vi "AlliGator FLI Dataset Loading Core.vi"(4 "Data Description":string, 5 "Control References":T4, 6 "Metadata":string, 7 "Image Type":string, 8 "error in (no error)":errorcluster, 9 "FLI Data File Information":T1, 10 "selected path":path, 11 "Data Value Reference in":refnum<data-value>) -> (0 "error out":errorcluster, 2 "Message":string, 3 "Data Value Reference out":refnum<data-value>)   [LabVIEW 2021, in "AlliGator Files.lvlib"]
doc: "Core VI handling loading the multiple gate images of a dataset as well as associated information and metadata. It dynamically calls a dataset-specific set of VIs to perform the actual loading."
uses:
  AlliGator Files.lvlib
  AlliGator Dataset Ctrl Refnums.ctl
  AlliGator Displayed Image.ctl
  AlliGator FLI Data File Information.ctl
  Phasor/Phasor Fluorescence Lifetime Parameters v3.ctl
  AlliGator FLI Dataset Type.ctl
  AlliGator Internal Variables v2.ctl
  <vilib>/vision/Image Controls.llb/IMAQ Image.ctl
  AlliGator Gate Image Set.ctl
  AlliGator Data Series Type.ctl
  AlliGator Dataset Channel.ctl
  AlliGator Gate Arithmetic.ctl
  Image/Named ROI Description.ctl
  AlliGator Decay Metadata v3.ctl
  AlliGator Decay Background Subtraction Info.ctl
  AlliGator Baseline Subtraction Method.ctl
  Graphs/XY Graph/XY Graph Plot Shift Parameters.ctl
  Graphs/XY Graph/XY Graph Plot Shift Method.ctl
  AlliGator Decay Extrapolation Parameters.ctl
  Phasor/Calibration Phasor (m, phi).ctl
  Phasor/Phasor Reference Series.ctl
  Phasor/Phasor Calibration Map v2.ctl
  Phasor/Phasor (g, s).ctl
  AlliGator Raw Phasor Plot Data v4.ctl
  Phasor/Phasor Standard Deviation Options.ctl
  AlliGator Phasor Multi-Harmonic Data.ctl
  Phasor/Phasor Harmonic Data.ctl
  AlliGator Decay Fit Options & Parameters v2.ctl
  Fits/IRF(X)PSED/Decay Fit Options v2.ctl
  Fits/Decay Convolution/Decay Model.ctl
  Fits/Residual Type.ctl
  Fits/IRF(X)PSED/Fit Weights Type.ctl
  Fits/Non-linear Fitting Method v2.ctl
  Fits/Fit Calculation Method.ctl
  Fits/Non-linear Fitting Algorithm.ctl
  AlliGator Decay Fit Parameter Constraints 2.ctl
  Fits/IRF(X)PSED/Decay Fit Parameters In List.ctl
  Fits/IRF(X)PSED/MLE Baseline Offset Type.ctl
  AlliGator Decay Preprocessing Parameters.ctl
  Fits/IRF(X)PSED/Decay Fit Parameters & Derived Quantities List.ctl
  AlliGator Parameter Maps Data.ctl
  AlliGator Image Pre-processing Parameters.ctl
  Arrays/Kernel Type.ctl
  Arrays/Smoothing Algorithm.ctl
  SwissSPAD/SwissSPAD Live_Image Display Options.ctl
  AlliGator Image Pre-processing Step.ctl
  AlliGator FLI Image Stack Action.ctl
  AlliGator Variables List.ctl
  AlliGator After Loading Dataset Information.ctl
  AlliGator ICCD-specific Information.ctl
  AlliGator Source Image.lvlib
  AlliGator HDF5.lvlib
  Time/Time.lvlib
  Arrays/Arrays.lvlib
  Strings/Strings.lvlib
  AlliGator GUI.lvlib
  GUI/GUI.lvlib
  Error/Error.lvlib
  AlliGator Dual-Channel Datasets.lvlib
  Image/Image.lvlib
  SwissSPAD/SwissSPAD Live.lvlib
  AlliGator Globals, Variables & Constants.lvlib
  Files/Files.lvlib
  Phasor/Phasor.lvlib
  AlliGator Decay Preprocessing.lvlib
  Graphs/XY Graph/XY Graph Add-Ons.lvlib
  AlliGator Phasor Graph.lvlib
  AlliGator Phasor Plot.lvlib
  Fits/Fits.lvlib
  AlliGator Decay Fit.lvlib
  AlliGator Decay Fit Parameter Map.lvlib
  AlliGator Internal Variables.lvlib
  AlliGator Settings.lvlib
panel:
  out "Dual-Channel Dataset":bool
  out "# created images":i32
  out "# Disposed Images":i32
  # "see the AlliGator License on the block diagram (Ctrl+E or Window:Show Block Diagram)"
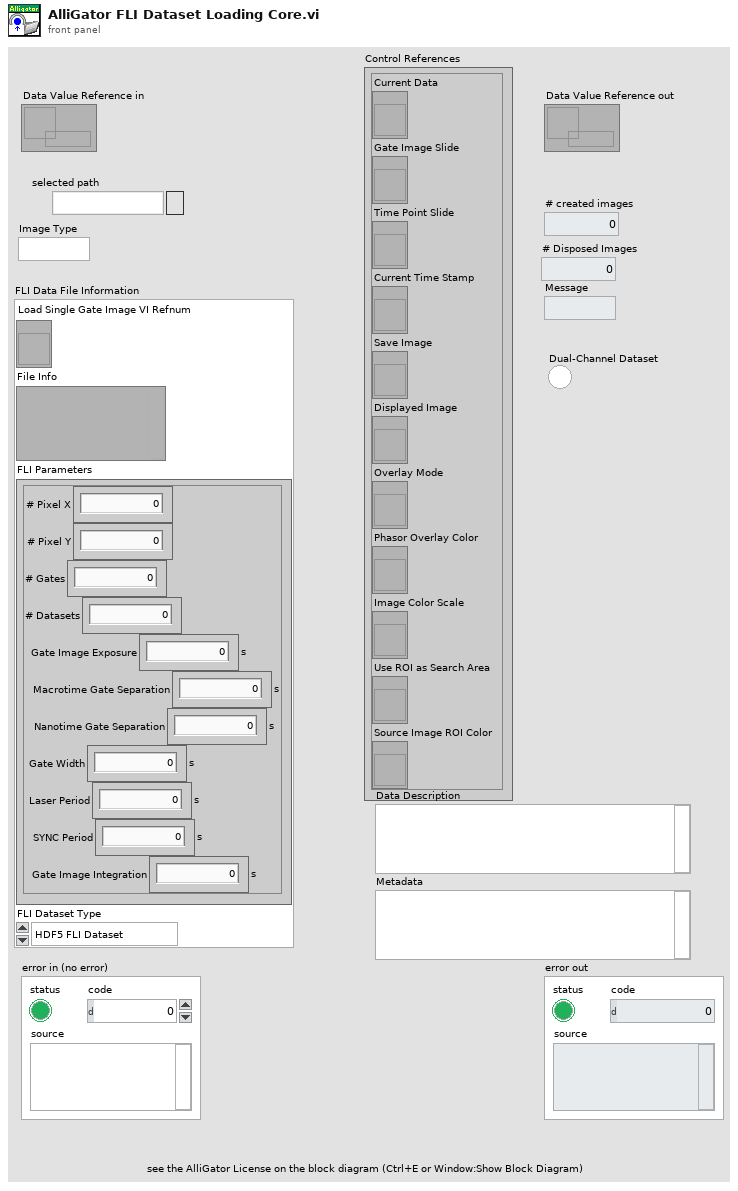
[diagram p1: front panel]
types:
  T1 = typedef "AlliGator HDF5.lvlib/AlliGator FLI Data File Information.ctl" = cluster{"Load Single Gate Image VI Refnum":refnum<vi>, "File Info":variant, "FLI Parameters":T2, "FLI Dataset Type":T3}
  T2 = typedef "Phasor.lvlib/Phasor Fluorescence Lifetime Parameters v3.ctl" = cluster{"# Pixel X":i32, "# Pixel Y":i32, "# Gates":i32, "# Datasets":i32, "Gate Image Exposure":dbl[unit], "Macrotime Gate Separation":dbl[unit], "Nanotime Gate Separation":dbl[unit], "Gate Width":dbl[unit], "Laser Period":dbl[unit], "SYNC Period":dbl[unit], "Gate Image Integration":dbl[unit]}
  T3 = typedef "AlliGator Files.lvlib/AlliGator FLI Dataset Type.ctl" = enum16{"HDF5 FLI Dataset", "Gate Image Folder", ".sdt FLI Dataset (Becker & Hickl)", ".ptu FLI Dataset (PicoQuant)", "SS1 FLI Dataset", "SS2 FLI Dataset", "I/m/phi Dataset", ".bin FLI Dataset (PicoQuant Binned)", ".bin FLI Dataset (Piccolo Binned)"}
  T4 = typedef "AlliGator GUI.lvlib/AlliGator Dataset Ctrl Refnums.ctl" = cluster{"Current Data":refnum<vi>, "Gate Image Slide":refnum<vi>, "Time Point Slide":refnum<vi>, "Current Time Stamp":refnum<vi>, "Save Image":refnum<vi>, "Displayed Image":refnum<vi>, "Overlay Mode":refnum<vi>, "Phasor Overlay Color":refnum<vi>, "Image Color Scale":refnum<vi>, "Use ROI as Search Area":refnum<vi>, "Source Image ROI Color":refnum<vi>}
  T5 = typedef "AlliGator Files.lvlib/AlliGator Image Pre-processing Parameters.ctl" = cluster{"Pile-up Correction":bool, "Pixel Well Capacity":u32, "Use Image Binning":bool, "X Bin":i32, "Y Bin":i32, "Use Image Smoothing":bool, "Kernel Type":T6, "Bin":i32, "Algorithm":T7, "Hot Pixel Removal":T8, "Dataset Scaling Factor":dbl, "Image Pre-processing Steps":T9[]}
  T6 = typedef "Arrays.lvlib/Kernel Type.ctl" = enum16{"Uniform", "Bilinear", "Gaussian"}
  T7 = typedef "Arrays.lvlib/Smoothing Algorithm.ctl" = enum16{"Rapid", "Thorough"}
  T8 = typedef "SwissSPAD Live.lvlib/SwissSPAD Live_Image Display Options.ctl" = cluster{"Remove Screamers":bool, "Delta":sgl, "Equalize Histogram":bool, "Percentile":sgl, "Hot Pixel Mask Image":path, "Use Hot Pixel Mask":bool}
  T9 = typedef "AlliGator Files.lvlib/AlliGator Image Pre-processing Step.ctl" = enum16{"Remove Screamers", "Pile-up Correction", "Binning", "Smoothing", "Rescaling", "Dead Left Column Correction"}
  T10 = typedef "AlliGator Source Image.lvlib/AlliGator Image Loading Options.ctl" = cluster{"Pixel Well Capacity":u32, "Pile-up Correction":bool, "Gate Step":i32, "Image Smoothing Options":T11, "Gates to Skip":T12, "File Background Subtraction":bool, "Background File Path":path, "Image Binning Options":T13, "# Gates":u32, "Gates to Keep":T14, "Define Gates to":bool, "Hot Pixel Removal":T8, "Dataset Scaling Factor":dbl, "Image Pre-processing Steps":T9[]}
  T11 = typedef "AlliGator Settings.lvlib/AlliGator Image Smoothing Options.ctl" = cluster{"Use Image Smoothing":bool, "Kernel Type":T6, "Bin":i32, "Algorithm":T7}
  T12 = typedef "AlliGator Decay Analysis.lvlib/AlliGator Gates to Skip.ctl" = cluster{"Start":u32, "End":u32}
  T13 = typedef "AlliGator Source Image.lvlib/AlliGator Image Binning Options.ctl" = cluster{"Use Image Binning":bool, "X Bin":i32, "Y Bin":i32}
  T14 = typedef "AlliGator Settings.lvlib/AlliGator Gates to Keep.ctl" = cluster{"First":u32, "Last":u32}
  T15 = typedef "AlliGator Settings.lvlib/AlliGator Gate Arithmetic.ctl" = enum16{"None", "INT-G2", "G2/INT*<INT>", "(1 - G2/INT)*<INT>"}
  T16 = typedef "AlliGator Dual-Channel Datasets.lvlib/AlliGator Dataset Channel.ctl" = enum16{"G2", "INT"}
  T17 = typedef "Image.lvlib/Image Characteristics.ctl" = cluster{"Calibration":T18, "File Type":string, "X Resolution":i32, "Y Resolution":i32, "File Data Type":i32, "Image Type":T20}
  T18 = typedef "Simple Grid Descriptor" = cluster{"X Step":sgl, "Y Step":sgl, "Unit":T19}
  T19 = typedef "Image Unit" = enum32{"Undefined", "Angström", "Micrometer", "Millimeter", "Centimeter", "Meter", "Kilometer", "Microinch", "Inch", "Feet", "Nautical miles", "Standard miles", "Steps"}
  T20 = typedef "Image Type" = u32
  T21 = typedef "AlliGator HDF5.lvlib/AlliGator FLI Image Stack Action.ctl" = enum16{"Init", "Get Image", "Close"}
  T22 = typedef "AlliGator Globals, Variables & Constants.lvlib/AlliGator Variables List.ctl" = enum16{"---- GUI ----", "GUI:Initialization Status", "GUI:State Indicators Refnum", "GUI:Original AlliGator Menu Items", "GUI:Current Action Loop State", "GUI:Script in progress", "GUI:Playback", "GUI:Loop Playback", "GUI:Search ROI Used", "GUI:Search ROI", "Decay Graph Max Legend Size", "Intensity Graph Max Legend Size", "Decay Statistics Graph Max Legend Size", "Phasor Graph Max Legend Size", "Phasor Ratio Graph Max Legend Size", "Lifetime Graph Max Legend Size", "---- Files ----", "Files:Export Dataset Frames as Individual Files", "Files:Show Batch Export Help Balloons", "Files:Frames in Dataset", "Files:ptu File Frame Start Indices", "Files:Current Frame in Dataset", "Files:Current Frame Timestamp", "Files:Dataset Loaded", "Files:Dataset Metadata", "Files:Dataset Channel", "Files:Dataset Data Description", "Files:Background Dataset Metadata", "Files:Background Dataset Channel", "Files:Background Dataset Data Description", "Files:Background File Subtraction", "Files:Background File Path", "Files:Background File Pile-up Correction", "Files:Background File Pixel Well Capacity", "Files:Background File Scaling Factor", "Files:Current Dataset Load Settings", "Files:Dataset Path", "Files:ICCD-specific Information", "Files:Macrotime Gate Separation", "------ Python Plugins ------", "Python Plugins:Information", "Python Plugins:Python Session", "Python Plugins:Valid Python Session?", "---- Source Image ----", "Source Image:ROIs", "Source Image:Current ROI", "Source Image:ROI Event Refnum", "X_Source Image Display Range", "X_Source Image Palette Information", "X_Type of Displayed Image", "X_Time Gate Slider", "Source Image:Palette List", "Source Image:Scale", "Source Image:ROI Overlay Color", "Source Image:Overlay to Erase", "Source Image:Is Displayed Image Accumulated", "Source Image:White Light Image Modified", "Source Image:Mask Image Modified", "---- Image Profile Window ----", "Image Profile:Window Event Refnum", "Image Profile:IntensityType", "Image Profile:Intensity Average Type", "Image Profile:Intensity-weighted SDV", "Image Profile:Box Profile Type", "Image Profile:Window Open", "Image Profile:Plotted Fit Parameter", "------ Phasor Graph -------", "Phasor Graph:Show Line", "---- Phasor Plot ---", "Phasor Plot:Parameters Changed", "Phasor Plot:FLI Dataset Modified since last Calculation", "Phasor Harmonics Data", "Selected Phasor Harmonics", "Phasor Harmonic Manager Event Refnum", "Phasor Plot:ROIs", "Phasor Plot:Current ROI", "Phasor Plot:ROI Event Refnum", "Phasor Plot:Image Reference Points", "Phasor Plot:Computed", "Phasor Plot:Palette Information", "Phasor Plot:Palette List", "Phasor Plot:Phasor Ratio Palette Information", "Phasor Plot:Phasor Ratio Palette List", "Phasor Plot:Image Scale", "Phasor Plot:Image Overlay to Erase", "Phasor Plot:Image Elements to Update", "Phasor Plot:Current Calculation Parameters", "Phasor Plot:Current Calibration Options", "Phasor Plot:Reset Cumulated Phasor Plot", "Phasor Plot:Reference 1", "Phasor Plot:Lifetime Reference 1", "Phasor Plot:Reference 1 Frequency", "Phasor Plot:Reference 2", "Phasor Plot:Lifetime Reference 2", "Phasor Plot:Reference 2 Frequency", "---- Decay Analysis ----", "Number of Selected Decays to Fit", "LS Fit Results", "LAR Fit Results", "BS Fit Results", "Last Decay Max - Min", "Best Fit Parameters", "Best Fit Parameter Names", "Actual Size X", "Actual Size Y", "Binning X", "Binning Y", "Actual # Gates", "Dataset Number", "Gates to...", "Gates Skipped", "Gates to keep", "Gate Step", "Gate Separation", "Reversed Gates", "Pile-up Correction", "Pixel Well Capacity", "Background Subtracted", "Background Subtraction Method", "Background Definition Range", "Background File (deprecated)", "Number of Dataset Accumulated", "Array of Accumulated Dataset Paths", "Do Averaged Datasets", "Destination File Path", "Process Plot Target", "Use 1/D as Phasor Frequency", "---- Decay Fit Parameter Map -----", "Decay Fit Parameter Map:Palette Information", "Decay Fit Parameter Map:Palette List", "------- Local Decay Window ---------", "Local Decay Graph Window:Event Refnum", "Local Decay Graph Window:Use normalized IRF for convolution", "----- Miscellaneous ----", "Misc:Skippable Dialog Windows Status"}
  T23 = typedef "AlliGator Internal Variables.lvlib/AlliGator Internal Variables v2.ctl" = cluster{"Displayed Image":T24, "White Light Image":T24, "Mask Image":T24, "ROI Mask Image":T24, "Current Dataset Images 1":T25, "Background Dataset Images 1":T25, "Current Dataset Images 2":T25, "Background Dataset Images 2":T25, "Current Dataset Arithmetic Images":T25, "Accumulated Dataset Images 1":T25, "Accumulated Dataset Images 2":T25, "Accumulated Dataset Arithmetic Images":T25, "Phasor Plot Image":T24, "Decay Fit Parameter Map Image":T24, "Single Data Point Path":path, "White Light Image Path":path, "Mask Image Path":path, "Time-Series Folder":path, "[Time-Series Paths]":path[], "Current Dataset":i32, "Single Dataset Type":T3, "Current Folder":string, "AlliGator Data Series Type":T26, "# Datasets":i32, "Dual-Channel Dataset":bool, "Selected Channel Name":string, "Dataset Channel":T16, "Channel Arithmetic":T15, "Dual-Channel Background Dataset":bool, "Background Channel":T16, "Dual-Channel Accumulated Dataset":bool, "Start Time":dbl, "[Time-Series Timestamps]":dbl[], "[Intensity Corrections]":dbl[], "Time Series Script":bool, "Type of Displayed Image":T27, "Gate Image Slide":u16, "# Gates":i32, "ROIs":T28[], "ROI Decay":cluster{"t Array":dbl[], "I Array":dbl[]}, "Valid Decay":bool, "Decay  Metadata":T30, "Reference Decay Plot Name":string, "Reference Decay":cluster{"t Array":dbl[], "I Array":dbl[]}, "Decay Shift Plot":cluster{"Time Stamps":dbl[], "Decay Shifts":dbl[]}, "[Decays Max Values]":sgl[], "[Decays Min Values]":sgl[], "Calibration Phasor":T36, "Calibration Phasor Series":T37, "Phasor Calibration Map":T38, "Calibration Map MD5 Digest":string, "Last Raw Phasor":T39, "Last Calibrated Phasor":T39, "Last Calibrated Phasor SDV":T39, "Phasor Graph:Phasor Plot":cluster{"g Array":dbl[], "s Array":dbl[]}, "Phasor Graph:Phasor SDV Plot":cluster{"g Array":dbl[], "s Array":dbl[]}, "[Phasor Graph:Raw Phasor Plots]":T40[], "Phasor Plot locked to Ref 1":i32, "[Phasor Plot(s) locked to Ref 1]":i32[], "[Phasor Plot(s) locked to Ref 2]":i32[], "[Pixel Phasors]":T39[], "[[Sum Image]]":dbl[][], "[[CSG Phasors]]":csg[][], "[[Valid Pixel?]]":bool[][], "I/m/phi Dataset":cluster{"I/m/phi Dataset?":bool, "Base Frequency":dbl[unit], "Harmonic Orders":u8[]}, "Multi Phasor Plot Data":T42, "Decay Fit Options & Parameters":T44, "Fit Options: Decay Preprocessing Parameters":T55, "Fit Options: Reference Decay":cluster{"t Array":dbl[], "I Array":dbl[]}, "Is Full Image Parameters Map":bool, "Is Single-Pixels Parameters Map":bool, "NLSF Parameters Map X Resolution":i32, "NLSF Parameters Map Y Resolution":i32, "[Single Decay Fit Parameters]":dbl[], "Fit Model":T46, "[[Multiple Decays Fit Parameters]]":dbl[][], "[[Multiple Decays Fit Parameter SDVs]]":dbl[][], "[[IRFs]]":dbl[][], "IRF Array Time Axis":dbl[], "Decay Array Time Axis":dbl[], "[Decay Fit Parameter Names]":T56[], "[[Phasor Ratios]]":dbl[][], "[[Average Lifetimes]]":dbl[][], "Amplitude Weighted Average Lifetime":bool, "[Decay Sum]":dbl[], "Parameter Maps":T57[], "[[User-defined Quantities]]":dbl[][], "User-defined Quantity":string}
  T24 = typedef "IMAQ Image.ctl" = refnum<image>
  T25 = typedef "AlliGator Internal Variables.lvlib/AlliGator Gate Image Set.ctl" = cluster{"SGL Image Max":T24, "SGL Image Sum":T24, "SGL Gate Images":T24[], "SGL Image Min":T24}
  T26 = typedef "AlliGator Files.lvlib/AlliGator Data Series Type.ctl" = enum16{"Not a Supported Series", "Gate Images Folder Series", "SwissSPAD 2 Dataset Series", "B&H FLI Dataset Series", "PicoQuant PTU FLI Dataset Series", "PicoQuant BIN FLI Dataset Series", "Piccolo hist BIN FLI Dataset Series", "HDF5 FLI Dataset Series"}
  T27 = typedef "AlliGator Source Image.lvlib/AlliGator Displayed Image.ctl" = enum16{"Single Gate", "Sum of All Gates", "Max of All Gates", "Min of All Gates", "-", "White Ligth Image", "Mask Image"}
  T28 = typedef "Image.lvlib/Named ROI Description.ctl" = cluster{"ROI Descriptor":T29, "ROI Name":string, "Overlay Color":u32}
  T29 = typedef "ROI Descriptor" = cluster{"Global Rectangle":i32[], "Contours":cluster{"ID":enum32{"External", "Internal"}, "Type":u32, "Coordinates":i32[]}[]}
  T30 = typedef "AlliGator Phasor Graph.lvlib/AlliGator Decay Metadata v3.ctl" = cluster{"ROI Descriptor":T29, "ROI Center":cluster{"X":i32, "Y":i32}, "Decay Background Subtraction Info":T31, "Decay Reverted":bool, "Decay Smoothened":bool, "Decay Straightened":bool, "Fitted Tau (Decay Straightening)":dbl, "Decay Shift Parameters":T33, "Decay Shifted":bool, "Decay Extrapolated":bool, "Decay Extrapolation Parameters":T35, "Decay Normalized":bool, "Fold Decay":bool, "# Folds":u32}
  T31 = typedef "AlliGator Decay Analysis.lvlib/AlliGator Decay Preprocessing.lvlib/AlliGator Decay Background Subtraction Info.ctl" = cluster{"Laser Period":dbl[unit], "Gate Duration":dbl[unit], "Baseline Subtraction Method":T32, "Background Definition Range":cluster{"Min Gate":dbl[unit], "Max Gate":dbl[unit]}, "Total Intensity w/o Bkgd Subtraction":dbl, "Bkgd-subtracted Intensity (exp)":dbl, "# Data Points":i32, "Background/Gate":dbl, "Fitted Lifetime":dbl[unit], "Bkgd-subtracted Intensity (theo)":dbl}
  T32 = typedef "AlliGator Decay Analysis.lvlib/AlliGator Decay Preprocessing.lvlib/AlliGator Baseline Subtraction Method.ctl" = enum16{"Mean", "Min", "Square Gated Single-Exponential", "File", "Constant"}
  T33 = typedef "XY Graph Add-Ons.lvlib/XY Graph Plot Shift Parameters.ctl" = cluster{"Type":T34, "Shift":dbl[unit], "Threshold":dbl, "Rotate":bool}
  T34 = typedef "XY Graph Add-Ons.lvlib/XY Graph Plot Shift Method.ctl" = enum16{"Default", "CFD", "Threshold", "Cross-Correlation"}
  T35 = typedef "AlliGator Decay Analysis.lvlib/AlliGator Decay Preprocessing.lvlib/AlliGator Decay Extrapolation Parameters.ctl" = cluster{"Additional Points":u32, "Head Fraction":dbl, "Fitted Tau":dbl, "Use Periodicity":bool, "Use Cursors":bool, "Tail Fraction":dbl}
  T36 = typedef "Phasor.lvlib/Calibration Phasor (m, phi).ctl" = cluster{"m":dbl, "phi":dbl, "Phasor Frequency":dbl[unit], "Reference Lifetime":dbl[unit]}
  T37 = typedef "Phasor.lvlib/Phasor Reference Series.ctl" = cluster{"m Array":dbl[], "phi Array":dbl[], "Phasor Frequency":dbl[unit], "Calibration Lifetime":dbl[unit]}
  T38 = typedef "Phasor.lvlib/Phasor Calibration Map v2.ctl" = cluster{"Phasor Frequency":dbl[unit], "Calibration Lifetime":dbl[unit], "ROI Centers":cluster{"X":i32, "Y":i32}[], "ROI Descriptors":T29[], "Map Resolution X":i32, "Map Resolution Y":i32, "z Array":cdb[]}
  T39 = typedef "Phasor.lvlib/Phasor (g, s).ctl" = cluster{"g":dbl, "s":dbl}
  T40 = typedef "AlliGator Phasor Graph.lvlib/AlliGator Raw Phasor Plot Data v4.ctl" = cluster{"Phasor Plot Name":string, "Raw Phasor Plot":T39[], "Phasor Frequency":dbl[unit], "[Decay Metadata]":T30[], "Raw Phasor Plot SDV":T39[], "Phasor SDV Options":T41, "[Calibration Phasor]":T36[]}
  T41 = typedef "Phasor.lvlib/Phasor Standard Deviation Options.ctl" = cluster{"Compute Estimated SDV":bool, "# Replicas":u32, "Use Estimated Average Phasor":bool}
  T42 = typedef "AlliGator Phasor Plot.lvlib/AlliGator Phasor Multi-Harmonic Data.ctl" = cluster{"Base Frequency":dbl[unit], "# Harmonics":u8, "Harmonic Orders":u8[], "Phasor Plot Settings Checksum":u64, "Phasor Harmonic Data Array":T43[]}
  T43 = typedef "Phasor.lvlib/Phasor Harmonic Data.ctl" = cluster{"Phasor Harmonic Name":string, "Phasor Plot Settings Checksum":u64, "Phasor Frequency":dbl[unit], "Base Frequency":dbl[unit], "Harmonic Order":u8, "Phasor Plot Parameters":string, "Phasor Array [[CSG]]":csg[][], "Dataset File Path":path}
  T44 = typedef "AlliGator Decay Fit Parameter Map.lvlib/AlliGator Decay Fit Options & Parameters v2.ctl" = cluster{"SYNC Period":dbl[unit], "Fit Options":T45, "Fit Parameter Constraints":T52[], "MLE Baseline Offset":dbl, "MLE Baseline Offset Type":T54}
  T45 = typedef "Fits.lvlib/Decay Fit Options v2.ctl" = cluster{"Show Fit Residuals":bool, "Fit Model":T46, "Residual Type":T47, "Max Decay Percentile":dbl, "Min Decay Percentile":dbl, "Show Full Decay":bool, "Weights":T48, "Fitting Method":T49, "Compute Parameter Uncertainties":bool, "Periodic Boundaries":bool, "Model Calculation":T50, "Period":dbl[unit], "Termination Criteria":cluster{"Max Iterations":i32, "Max Function Calls":i32, "Max Time":dbl[unit], "Function Tolerance":dbl, "Parameter Tolerance":dbl, "Gradient Tolerance":dbl, "Min Lambda":dbl, "Max Lambda":dbl, "Initial Tick Count":u32}, "Offset Resolution":dbl[unit], "Use Local IRF":bool, "Fitting Algorithm":T51}
  T46 = typedef "Fits.lvlib/Decay Model.ctl" = enum16{"1-Exponential", "2-Exponentials"}
  T47 = typedef "Fits.lvlib/Residual Type.ctl" = enum16{"Standard", "Normalized", "Reduced"}
  T48 = typedef "Fits.lvlib/Fit Weights Type.ctl" = enum16{"Unweighted", "1/Variance", "Best of All"}
  T49 = typedef "Fits.lvlib/Non-linear Fitting Method v2.ctl" = enum16{"Least Square", "Least Absolute Residual", "Bisquare", "MLE", "-", "Best of All"}
  T50 = typedef "Fits.lvlib/Fit Calculation Method.ctl" = enum16{"Simulation", "Convolution", "Integration"}
  T51 = typedef "Fits.lvlib/Non-linear Fitting Algorithm.ctl" = enum16{"Levenberg-Marquardt", "Trust-Region Dogleg"}
  T52 = typedef "AlliGator Decay Analysis.lvlib/AlliGator Decay Fit.lvlib/AlliGator Decay Fit Parameter Constraints 2.ctl" = cluster{"Fit Parameter":T53, "Min Value":dbl, "Max Value":dbl, "Global":bool, "Used":bool}
  T53 = typedef "Fits.lvlib/Decay Fit Parameters In List.ctl" = enum16{"Offset", "Baseline", "A_1", "tau_1", "A_2", "tau_2"}
  T54 = typedef "Fits.lvlib/MLE Baseline Offset Type.ctl" = enum32{"Absolute", "Percentage"}
  T55 = typedef "AlliGator Decay Analysis.lvlib/AlliGator Decay Preprocessing.lvlib/AlliGator Decay Preprocessing Parameters.ctl" = cluster{"Background Subtraction":bool, "Straighten Decay":bool, "Reverse Gates":bool, "1-Normalized Decay":bool, "Smoothen Decay":bool, "Smoothing Parameter":dbl, "Shift Decay":bool, "Decay Shift Parameters":T33, "Extrapolate Decay":bool, "Additional Points":u32, "Head Fraction":dbl, "Pixel-Normalize Decay":bool, "Use Periodicity":bool, "Use Cursors":bool, "Tail Fraction":dbl, "Use Decay Pre-Processing":bool, "Fold Decay":bool, "# Folds":u32, "[0-1]-Normalized Decay":bool}
  T56 = typedef "Fits.lvlib/Decay Fit Parameters & Derived Quantities List.ctl" = enum16{"Offset", "Baseline", "A_1", "tau_1", "A_2", "tau_2", "<tau>_a", "f1_a", "f2_a", "<tau>_i", "f1_i", "f2_i", "-", "R^2", "Chi^2"}
  T57 = typedef "AlliGator Parameter Maps Data.ctl" = cluster{"Map Set Name":string, "[Parameter Names]":string[], "[[Parameters]]":dbl[][], "[[Parameter SDVs]]":dbl[][], "Decay Array Time Axis":dbl[], "[[IRFs]]":dbl[][], "IRF Array Time Axis":dbl[]}
  T58 = typedef "AlliGator Files.lvlib/AlliGator ICCD-specific Information.ctl" = cluster{"V MCP":dbl[unit], "X Hardware Binning":dbl, "Y Hardware Binning":dbl, "Gate Image Integration":dbl[unit], "Laser Power":dbl[unit]}
  T59 = typedef "AlliGator Files.lvlib/AlliGator After Loading Dataset Information.ctl" = cluster{"Nanotime Gate Separation":dbl[unit], "Gate Width":dbl[unit], "Laser Period":dbl[unit], "Data Description":string, "# Pixel X":i32, "# Pixel Y":i32, "Gates to Use":cluster{"Start":u32, "End":u32}, "Gate Step":i32, "SYNC Period":dbl[unit], "X Binning":i32, "Y Binning":i32, "Gates to":bool, "Metadata":string, "Gate Image Exposure":dbl[unit], "Gate Image Integration":dbl[unit], "Macrotime Gate Separation":dbl[unit], "ICCD-specific Information":T58}
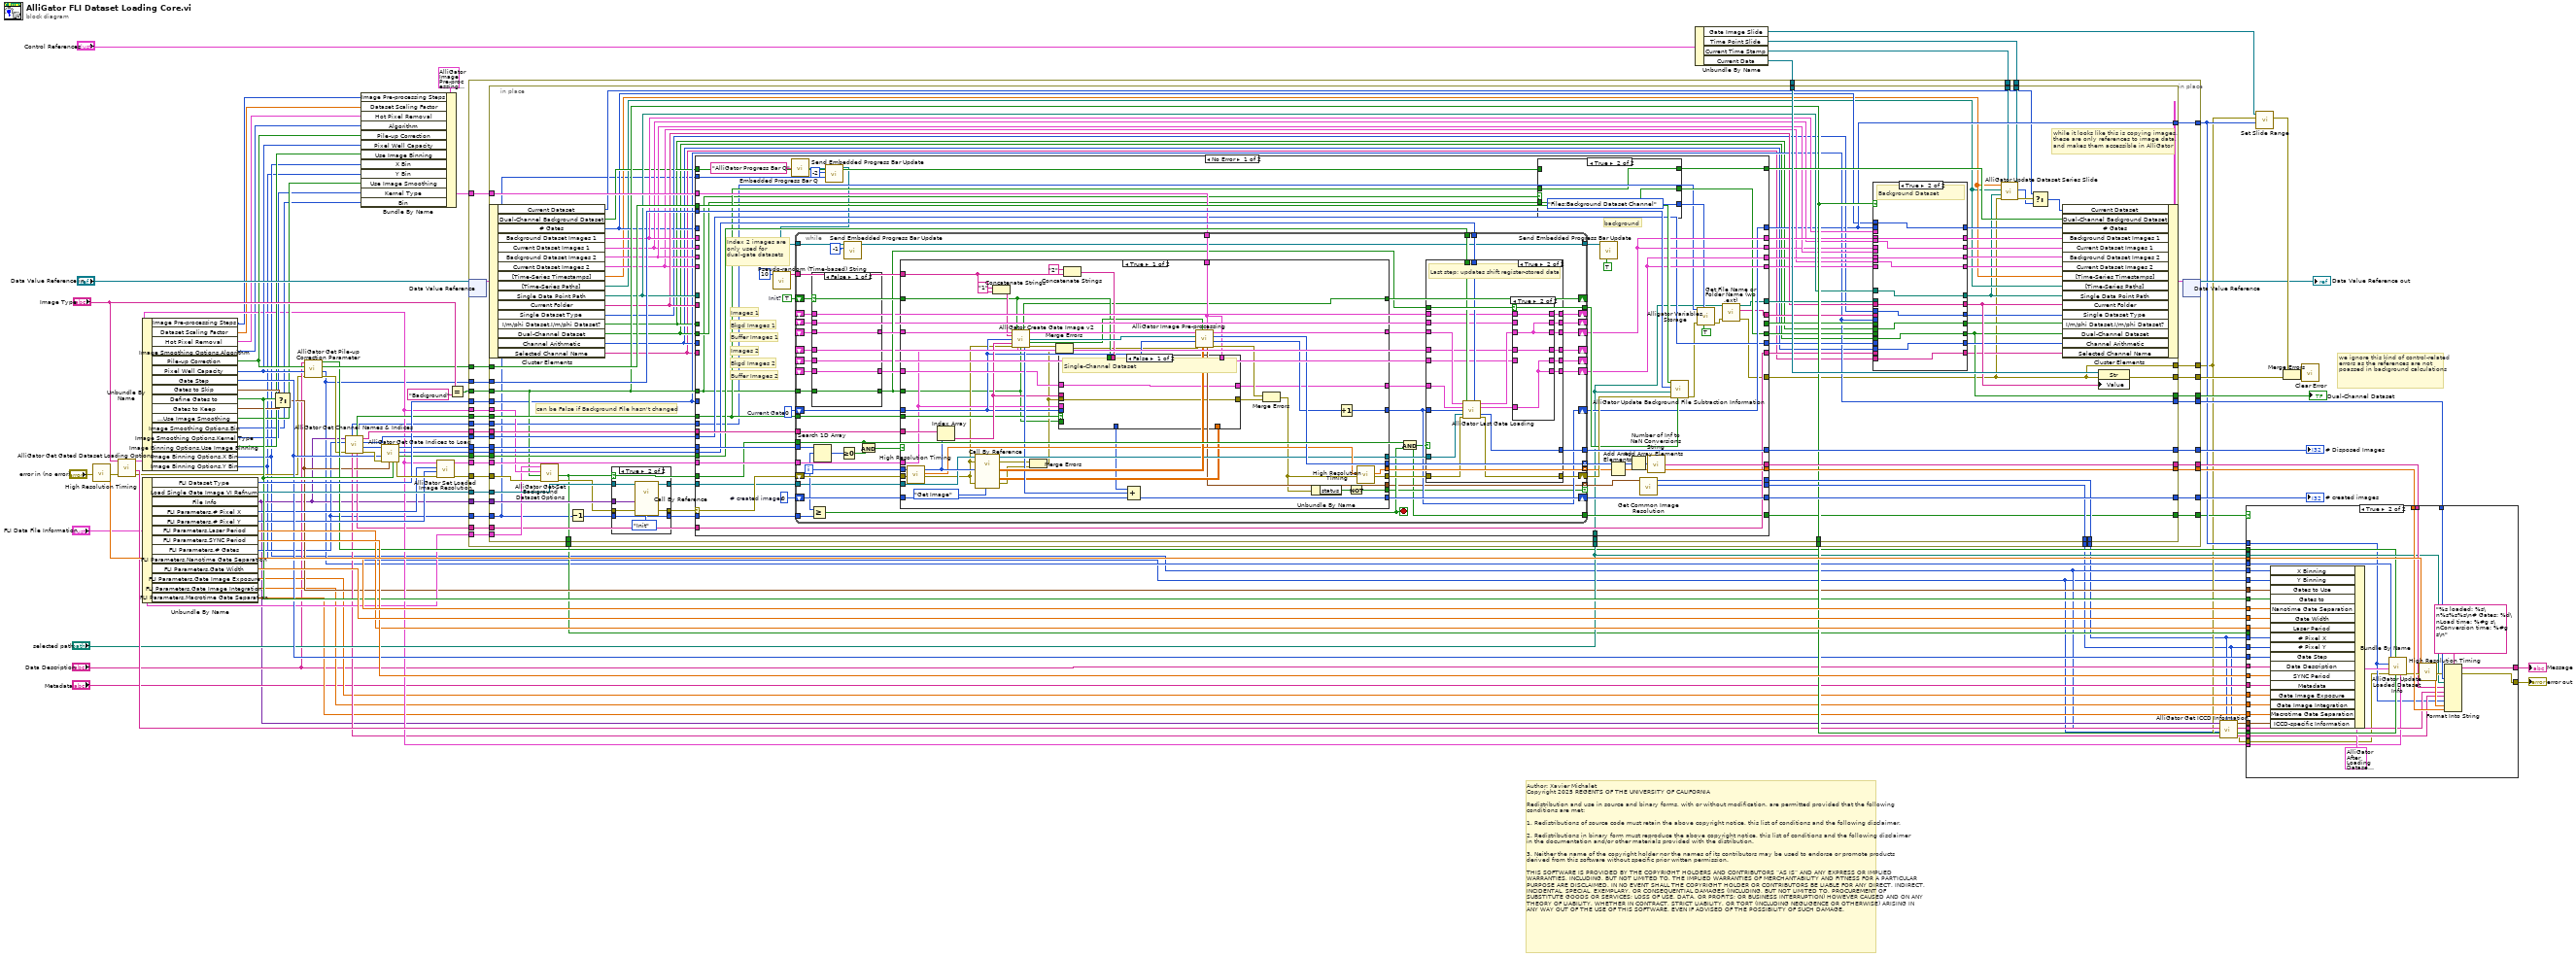
[diagram p0: block diagram]
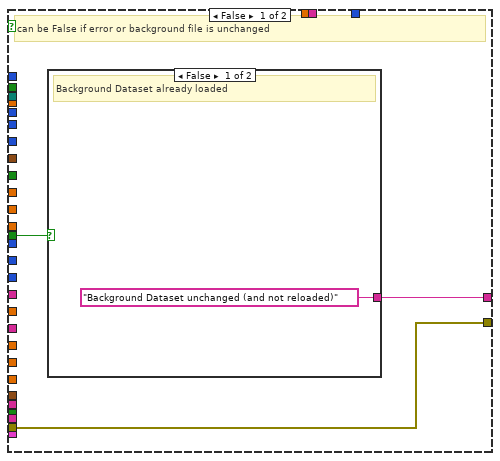
[diagram p2: hidden frame]
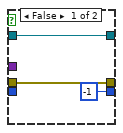
[diagram p5: hidden frame]
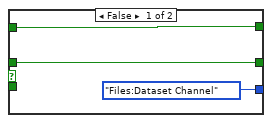
[diagram p6: hidden frame]
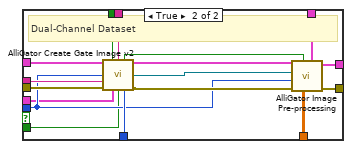
[diagram p9: hidden frame]
diagram:
  # "Author: Xavier Michalet\nCopyright 2025 REGENTS OF THE UNIVERSITY OF CALIFORNIA\n\nRedistribution and use in source and binary forms, with or without modification, are permitted provided that the following conditions are met:\n\n1. Redistributions of source code must retain the above copyright notice, this list of conditions and the following disclaimer.\n\n2. Redistributions in binary form must reproduce the above copyright notice, this list of conditions and the following disclaimer in the documentation and/or other materials provided with the distribution.\n\n3. Neither the name of the copyright holder nor the names of its contributors may be used to endorse or promote products derived from this software without specific prior written permission.\n\nTHIS SOFTWARE IS PROVIDED BY THE COPYRIGHT HOLDERS AND CONTRIBUTORS “AS IS” AND ANY EXPRESS OR IMPLIED WARRANTIES, INCLUDING, BUT NOT LIMITED TO, THE IMPLIED WARRANTIES OF MERCHANTABILITY AND FITNESS FOR A PARTICULAR PURPOSE ARE DISCLAIMED. IN NO EVENT SHALL THE COPYRIGHT HOLDER OR CONTRIBUTORS BE LIABLE FOR ANY DIRECT, INDIRECT, INCIDENTAL, SPECIAL, EXEMPLARY, OR CONSEQUENTIAL DAMAGES (INCLUDING, BUT NOT LIMITED TO, PROCUREMENT OF SUBSTITUTE GOODS OR SERVICES; LOSS OF USE, DATA, OR PROFITS; OR BUSINESS INTERRUPTION) HOWEVER CAUSED AND ON ANY THEORY OF LIABILITY, WHETHER IN CONTRACT, STRICT LIABILITY, OR TORT (INCLUDING NEGLIGENCE OR OTHERWISE) ARISING IN ANY WAY OUT OF THE USE OF THIS SOFTWARE, EVEN IF ADVISED OF THE POSSIBILITY OF SUCH DAMAGE."
  # "we ignore this kind of control-related errors as the references are not poassed in background calculations"
  n1 = call "High Resolution Timing.vi"("Error In"="error in (no error)") -> ("elapsed (relative) seconds"=w89:dbl, "Error Out"=w90:errorcluster)  [unwired: 16 in, 1 out]
  n2 = call "AlliGator Get Gated Dataset Loading Options.vi"("error in (no error)"=w90, "Image Type"="Image Type") -> ("error out"=w16:errorcluster, "Dataset Loading Options string"=w52:string, "Dataset Loading Options"=w32:T10)  [unwired: 6 in, 1 out]
  n3 = Unbundle By Name(w32) -> ("Image Pre-processing Steps"=w12:T9[], "Dataset Scaling Factor"=w13:dbl, "Hot Pixel Removal"=w11:T8, "Image Smoothing Options.Algorithm"=w10:T7, "Pile-up Correction"=w43:bool, "Pixel Well Capacity"=w42:u32, "Gate Step"=w65:i32, "Gates to Skip"=w64:T12, "Define Gates to"=w66:bool, "Gates to Keep"=w63:T14, "Image Smoothing Options.Use Image Smoothing"=w40:bool, "Image Smoothing Options.Bin"=w38:i32, "Image Smoothing Options.Kernel Type"=w39:T6, "Image Binning Options.Use Image Binning"=w41:bool, "Image Binning Options.X Bin"=w4:i32, "Image Binning Options.Y Bin"=w3:i32)
  n4 = Unbundle By Name("FLI Data File Information") -> ("FLI Dataset Type"=w80:T3, "Load Single Gate Image VI Refnum"=w77:refnum<vi>, "File Info"=w9:variant, "FLI Parameters.# Pixel X"=w50:i32, "FLI Parameters.# Pixel Y"=w51:i32, "FLI Parameters.Laser Period"=w73:dbl[unit], "FLI Parameters.SYNC Period"=w74:dbl[unit], "FLI Parameters.# Gates"=w14:i32, "FLI Parameters.Nanotime Gate Separation"=w75:dbl[unit], "FLI Parameters.Gate Width"=w76:dbl[unit], "FLI Parameters.Gate Image Exposure"=w27:dbl[unit], "FLI Parameters.Gate Image Integration"=w26:dbl[unit], "FLI Parameters.Macrotime Gate Separation"=w24:dbl[unit])
  n5 = Select(t=w64, s=w66, f=w63) -> (s? t:f=w29:T14)
  n6 = call "AlliGator Get Pile-up Correction Parameter.vi"("error in (no error)"=w16, "Pixel Well Capacity in"=w42, "Pile-up Correction in"=w43, "Data Information"="Data Description") -> ("error out"=w15:errorcluster, "Pixel Well Capacity out"=w5:u32, "Pile-up Correction out"=w46:bool, "Pile-up Correction (already) applied?"=w44:bool)  [unwired: 4 in]
  n7 = call "AlliGator Get Channel Names & Indices.vi"("error in (no error)"=w15, "# Gates"=w14, "File Info"=w9) -> ("error out"=w83:errorcluster, "Gate Indices"=w82:i32[], "Channel Arithmetic"=w34:T15, "Gate Image Names"=w81:string[], "Selected Channel Name"=w28:string, "Dual-Channel Dataset"=w35:bool, "Selected Channel Message"=w30:string, "Dataset Channel"=w25:T16)  [unwired: 1 in]
  n8 = Bundle By Name(cluster=T5 {"Pile-up Correction"=FALSE, "Pixel Well Capacity"=0, "Use Image Binning"=FALSE, "X Bin"=0, "Y Bin"=0, "Use Image Smoothing"=FALSE, "Kernel Type"=enum."Uniform", "Bin"=0, "Algorithm"=enum."Rapid", "Hot Pixel Removal"={"Remove Screamers"=FALSE, "Delta"=0.0, "Equalize Histogram"=FALSE, "Percentile"=0.0, "Hot Pixel Mask Image"=path "", "Use Hot Pixel Mask"=FALSE}, "Dataset Scaling Factor"=0.0, "Image Pre-processing Steps"=[]}, "Image Pre-processing Steps"=w12, "Dataset Scaling Factor"=w13, "Hot Pixel Removal"=w11, "Algorithm"=w10, "Pile-up Correction"=w43, "Pixel Well Capacity"=w42, "Use Image Binning"=w41, "X Bin"=w4, "Y Bin"=w3, "Use Image Smoothing"=w40, "Kernel Type"=w39, "Bin"=w38) -> (w36:T5)
  n9 = call "AlliGator Get Gate Indices to Load.vi"("Gates to?"=w66, "Gates to Use"=w29, "Error In"=w83, "Gate Step"=w65, "Gate Indices in"=w82) -> ("Error Out"=w84:errorcluster, "Gates across boundaries?"=w68:bool, "Split Index"=w67:u32, "Gate Indices out"=w62:i32[])  [unwired: 3 in]
  n10 = call "AlliGator Set Loaded Image Resolution.vi"("Error In"=w84, "Image Y"=w51, "Image X"=w50, "Image Loading Options"=w32) -> ("Error Out"=w53:errorcluster, "Image Characteristics"=w49:T17)  [unwired: 6 in]
  n11 = Equal?(x="Image Type", y="Background" ("x")) -> (x = y?=w70:bool)
  n12 = Unbundle By Name("Control References") -> ("Gate Image Slide"=w56:refnum<vi>, "Time Point Slide"=w17:refnum<vi>, "Current Time Stamp"=w18:refnum<vi>, "Current Data"=w55:refnum<vi>)
  n13 = in-place {
    in-place-border: [w130] -> w85
    in-place-border: w81 -> [w129]
    in-place-border: w62 -> [w128]
    in-place-border: [w127] -> w48
    in-place-border: w49 -> [w126]
    in-place-border: [w125] -> w86
    in-place-border: w14 -> [w124]
    in-place-border: w46 -> [w123]
    in-place-border: [w122] -> w7
    in-place-border: w5 -> [w121]
    in-place-border: w53 -> [w120]
    in-place-border: "selected path" -> [w119]
    in-place-border: w55 -> [w116]
    in-place-border: [w115] -> w21
    in-place-border: [w114] -> w60
    in-place-border: w67 -> [w113]
    in-place-border: w68 -> [w112]
    in-place-border: w70 -> [w111]
    in-place-border: [w110] -> w72
    in-place-border: w9 -> [w109]
    in-place-border: w77 -> [w108]
    in-place-border: [w107] -> w78
    in-place-border: [w106] -> w79
    in-place-border: w80 -> [w105]
    in-place-border: w36 -> [w104]
    in-place-border: w35 -> [w103]
    in-place-border: w34 -> [w102]
    in-place-border: [w101] -> w33
    in-place-border: w32 -> [w100]
    in-place-border: "FLI Data File Information" -> [w99]
    in-place-border: w28 -> [w98]
    in-place-border: [w97] -> w2
    in-place-border: [w96] -> w1
    in-place-border: w25 -> [w95]
    in-place-border: [w94] -> w20
    in-place-border: [w93] -> w19
    in-place-border: w18 -> [w92]
    in-place-border: w17 -> [w91]
    n14 = in-place-dvr #1("Data Value Reference in") -> (w118:T23)  [unwired: 1 out]
    n15 = in-place {
      in-place-border: [w212] -> w130
      in-place-border: w129 -> [w211]
      in-place-border: w128 -> [w210]
      in-place-border: [w209] -> w127
      in-place-border: w126 -> [w208]
      in-place-border: [w207] -> w125
      in-place-border: w124 -> [w131]
      in-place-border: w123 -> [w206]
      in-place-border: [w139] -> w122
      in-place-border: w121 -> [w205]
      in-place-border: w120 -> [w198]
      in-place-border: w119 -> [w204]
      in-place-border: w116 -> [w203]
      in-place-border: [w151] -> w115
      in-place-border: [w202] -> w114
      in-place-border: w113 -> [w201]
      in-place-border: w112 -> [w200]
      in-place-border: w111 -> [w181]
      in-place-border: [w181] -> w110
      in-place-border: w109 -> [w197]
      in-place-border: w108 -> [w196]
      in-place-border: [w156] -> w107
      in-place-border: [w194] -> w106
      in-place-border: w105 -> [w156]
      in-place-border: w104 -> [w193]
      in-place-border: w103 -> [w189]
      in-place-border: w102 -> [w192]
      in-place-border: [w160] -> w101
      in-place-border: w100 -> [w188]
      in-place-border: w99 -> [w187]
      in-place-border: w98 -> [w186]
      in-place-border: [w185] -> w97
      in-place-border: [w184] -> w96
      in-place-border: w95 -> [w182]
      in-place-border: [w144] -> w94
      in-place-border: [w143] -> w93
      in-place-border: w92 -> [w138]
      in-place-border: w91 -> [w137]
      # "can be False if Background File hasn't changed"
      # "while it looks like this is copying images,\nthese are only references to image data, \nand makes them accessible in AlliGator"
      n16 = in-place-cluster #2(w118) -> ("Current Dataset"=w133:i32, "Dual-Channel Background Dataset"=w152:bool, "# Gates"=w149:i32, "Background Dataset Images 1"=w175:T25, "Current Dataset Images 1"=w169:T25, "Background Dataset Images 2"=w172:T25, "Current Dataset Images 2"=w166:T25, "[Time-Series Timestamps]"=w142:dbl[], "[Time-Series Paths]"=w141:path[], "Single Data Point Path"=w180:path, "Current Folder"=w176:string, "Single Dataset Type"=w155:T3, "I/m/phi Dataset.I/m/phi Dataset?"=w148:bool, "Dual-Channel Dataset"=w147:bool, "Channel Arithmetic"=w146:T15, "Selected Channel Name"=w145:string)
      n17 = call "AlliGator Get-Set Background Dataset Options.vi"("error in (no error)"=w198, "Background Dataset"=w181, "Image Loading Options"=w188, "FLI Data File Information"=w187) -> ("error out"=w191:errorcluster, "Load Dataset?"=w143:bool)  [unwired: 6 in]
      n18 = Decrement(x=w131) -> (x-1=w132:i32)
      n19 = case shown="True" w143 {
        tunnel: [w238 w245] -> w199
        tunnel: w197 -> [_ w244]
        tunnel: w196 -> [w239 w243]
        tunnel: [w239 w242] -> w195
        tunnel: w191 -> [w238 w241]
        tunnel: w132 -> [_ w240]
        tunnel: [-1 w240] -> w190
        frame False {
        }
        frame True {
          n20 = call-by-ref "?"(reference=w243, "Action"=AlliGator_FLI_Image_Stack_Action."Init", "error in (no error)"=w241, "File Info"=w244) -> (reference out=w242:refnum<vi>, "error out"=w245:errorcluster)  [unwired: 7 in, 3 out]
        }
      }
      n21 = case shown="No Error" w199 {
        selector: w199 -> [w294 w502]
        tunnel: [w278 _] -> w212
        tunnel: w211 -> [w300 _]
        tunnel: w210 -> [w299 _]
        tunnel: [w296 _] -> w209
        tunnel: w208 -> [w295 _]
        tunnel: w204 -> [w258 _]
        tunnel: [w293 _] -> w207
        tunnel: w205 -> [w286 _]
        tunnel: w206 -> [w287 _]
        tunnel: w190 -> [w291 _]
        tunnel: [w254 w502] -> w139
        tunnel: [w275 w501] -> w151
        tunnel: [w279 w500] -> w164
        tunnel: [w257 w499] -> w179
        tunnel: [w256 w498] -> w178
        tunnel: w180 -> [_ w499]
        tunnel: w176 -> [_ w498]
        tunnel: w166 -> [_ w500]
        tunnel: w149 -> [_ w501]
        tunnel: w181 -> [w266 _]
        tunnel: w175 -> [_ w497]
        tunnel: [w280 w497] -> w174
        tunnel: w148 -> [_ w496]
        tunnel: [_ w496] -> w159
        tunnel: w201 -> [w290 _]
        tunnel: w200 -> [w289 _]
        tunnel: w195 -> [w285 _]
        tunnel: [w283 _] -> w194
        tunnel: w156 -> [_ _]
        tunnel: w193 -> [w282 _]
        tunnel: w169 -> [_ w495]
        tunnel: w172 -> [_ w494]
        tunnel: w189 -> [w269 _]
        tunnel: w192 -> [w270 _]
        tunnel: [w280 w495] -> w167
        tunnel: [w279 w494] -> w170
        tunnel: w143 -> [w277 _]
        tunnel: w147 -> [w267 w493]
        tunnel: [w268 w493] -> w161
        tunnel: w146 -> [_ w492]
        tunnel: w145 -> [_ w491]
        tunnel: [w270 w492] -> w163
        tunnel: [w274 w491] -> w154
        tunnel: w186 -> [w274 _]
        tunnel: [w272 _] -> w185
        tunnel: [w271 _] -> w184
        tunnel: w152 -> [w265 w490]
        tunnel: [w264 w490] -> w183
        tunnel: w182 -> [w260 _]
        tunnel: [w259 _] -> w144
        tunnel: w131 -> [w247 _]
        frame No Error {
          w302 = 0  # Current Gate
          w303 = TRUE  # Init?
          w301 = 0  # # created images
          # "Index 2 images are only used for dual-gate datasets"
          # "Images 2"
          # "Bkgd Images 2"
          # "Buffer Images 2"
          # "Images 1"
          # "Bkgd Images 1"
          # "Buffer Images 1"
          n22 = call "Pseudo-random (Time-based) String.vi"("Length (10)"=u32 10) -> ("result string"=w288:string)  [unwired: 9 in, 1 out]
          n23 = call "Embedded Progress Bar Q.vi"("Progress Bar Queue Name"="AlliGator Progress Bar Q") -> ("Progress Bar Queue"=w251:refnum<queue>)  [unwired: 6 in]
          n24 = call "Send Embedded Progress Bar Update.vi"("Max Iterations N"=w247, "Current Iteration i (i or -1: standard or || iteration; 0 or -2: first standard or || iteration)"=-2 ("Current Iteration i (i or -1: standard or || iteration; 0 or -2: first standard or || iteration)"), "Progress Bar Queue in"=w251) -> ("Progress Bar Queue out"=w250:refnum<queue>)  [unwired: 7 in, 1 out]
          n25 = while {
            tunnel: w300 -> [w354]
            shift-right: [w335] -> w292
            shift-left: w294 -> [w343]
            shift-right: [w346] -> _
            shift-left: w303 -> [w356]
            shift-right: [w333] -> w275
            shift-left: w302 -> [w355]
            shift-right: [w344] -> w278
            shift-left: w301 -> [w351]
            shift-right: [w349] -> _
            shift-left: _ -> [w323]
            tunnel: w299 -> [w362]
            tunnel: w288 -> [w358]
            tunnel: [w345] -> w298 mode=indexing
            shift-right: [w348] -> _
            shift-left: _ -> [w322]
            shift-right: [w347] -> w280
            shift-left: _ -> [w359]
            tunnel: w266 -> [w360]
            tunnel: w295 -> [w352]
            tunnel: [w361] -> w293
            tunnel: w291 -> [w341]
            tunnel: w290 -> [w340]
            tunnel: w289 -> [w339]
            tunnel: w285 -> [w338]
            tunnel: [w337] -> w284 mode=indexing
            tunnel: w282 -> [w332]
            shift-right: [w324] -> _
            shift-left: _ -> [w321]
            shift-right: [w326] -> _
            shift-left: _ -> [w320]
            shift-right: [w325] -> w279
            shift-left: _ -> [w331]
            tunnel: w269 -> [w329]
            tunnel: [w327] -> w281
            tunnel: w277 -> [w316]
            tunnel: [w315] -> w273 mode=indexing if=w314
            tunnel: [w313] -> w259
            tunnel: w250 -> [w311]
            tunnel: [w310] -> w248
            i -> [w342]
            stop <- w317 stop-if-true
            n26 = Greater Or Equal?(x=w342, y=w341) -> (x >= y?=w317:bool)
            n27 = case shown="False" w356 {
              tunnel: w360 -> [w478 w485]
              tunnel: [w478 w485] -> w327
              tunnel: w323 -> [_ w482]
              tunnel: w322 -> [_ w483]
              tunnel: w359 -> [w477 _]
              tunnel: [w477 w484] -> w357
              tunnel: w321 -> [_ w481]
              tunnel: w320 -> [_ w479]
              tunnel: [w476 w480] -> w330
              tunnel: w331 -> [w476 _]
              frame False {
              }
              frame True {
                # "Select which images to update"
                n28 = case shown="False" w485 {
                  tunnel: [w487 w489] -> w484
                  tunnel: w483 -> [_ w489]
                  tunnel: w482 -> [w487 _]
                  tunnel: w481 -> [w486 _]
                  tunnel: [w486 w488] -> w480
                  tunnel: w479 -> [_ w488]
                  frame False {
                  }
                  frame True {
                  }
                }
              }
            }
            n29 = Search 1D Array(1D array=w362, element=w342) -> (index of element=w353:i32)  [unwired: 1 in]
            n30 = Greater Or Equal To 0?(x=w353) -> (x >= 0?=w319:bool)
            n31 = call "Send Embedded Progress Bar Update.vi"("Current Iteration i (i or -1: standard or || iteration; 0 or -2: first standard or || iteration)"=-1 ("Current Iteration i (-1: || iteration, -2: first || iteration)"), "Progress Bar Queue in"=w311) -> ("Progress Bar Queue out"=w310:refnum<queue>)  [unwired: 8 in, 1 out]
            n32 = Compound Arithmetic op=AND(w316, w319) -> (w318:bool)
            n33 = case shown="True" w318 {
              tunnel: w343 -> [w441 w475]
              tunnel: w352 -> [w415 _]
              tunnel: w354 -> [w449 _]
              tunnel: w356 -> [w414 w473]
              tunnel: [w405 w473] -> w346
              tunnel: w355 -> [w417 w470]
              tunnel: [w436 w471] -> w350
              tunnel: w351 -> [w447 w474]
              tunnel: [w448 w474] -> w344
              tunnel: [w439 w475] -> w336
              tunnel: w358 -> [w424 _]
              tunnel: [w446 _] -> w345
              tunnel: w327 -> [w406 _]
              tunnel: w342 -> [w444 _]
              tunnel: w357 -> [w430 w471]
              tunnel: w338 -> [w443 w472]
              tunnel: [w437 _] -> w337
              tunnel: [w435 w472] -> w334
              tunnel: [w404 w470] -> w333
              tunnel: w332 -> [w420 _]
              tunnel: w330 -> [w427 w469]
              tunnel: w329 -> [w416 _]
              tunnel: [w407 w469] -> w328
              tunnel: [w403 _] -> w315
              tunnel: [w400 _] -> w314
              frame True {
                n34 = call "High Resolution Timing.vi"("Error In"=w441) -> ("elapsed (relative) seconds"=w438:dbl, "Error Out"=w412:errorcluster)  [unwired: 16 in, 1 out]
                n35 = Index Array(array=w449, index=w444) -> (element=w426:string)
                n36 = call-by-ref "?"(reference=w443, error in=w412, "Action"=AlliGator_FLI_Image_Stack_Action."Get Image", 8:"error in (no error)"=w412, "Gate Index"=w444) -> (reference out=w435:refnum<vi>, error out=w411:errorcluster, 0:"error out"=w413:errorcluster, "Data 2"=w429:sgl[][], "Data 1"=w442:sgl[][])  [unwired: 6 in]
                n37 = Concatenate Strings("1" ("string"), w424) -> (w425:string)
                n38 = call "AlliGator Create Gate Image v2.vi"("Dataset Images in"=w430, "Init?"=w414, "Prefix"=w425, "Current Gate"=w417, "Gate Name"=w426, "error in (no error)"=w412, "Image Characteristics"=w415, "Background Dataset"=w406) -> ("Init?"=w405:bool, "Dataset Images out"=w431:T25, "New Gate Image Refnum"=w432:T24, "Buffer Image available?"=w419:bool, "Number of Created Images"=w433:i32, "error out"=w410:errorcluster)  [unwired: 2 in]
                n39 = Merge Errors(w411, w413) -> (w408:errorcluster)
                n40 = Merge Errors(w410, w408) -> (w409:errorcluster)
                n41 = Concatenate Strings("2" ("string"), w424) -> (w422:string)
                n42 = case shown="False" w416 {
                  tunnel: w429 -> [_ w468]
                  tunnel: [w451 w467] -> w428
                  tunnel: w427 -> [w450 w466]
                  tunnel: w426 -> [_ w465]
                  tunnel: w408 -> [w451 w464]
                  tunnel: w414 -> [_ w463]
                  tunnel: w422 -> [_ w462]
                  tunnel: w420 -> [_ w459]
                  tunnel: [_ w457] -> w418
                  tunnel: w417 -> [_ w455]
                  tunnel: w415 -> [_ w454]
                  tunnel: [w450 w453] -> w407
                  tunnel: w406 -> [_ w452]
                  frame False {
                    # "Single-Channel Dataset"
                  }
                  frame True {
                    # "Dual-Channel Dataset"
                    n43 = call "AlliGator Create Gate Image v2.vi"("Dataset Images in"=w466, "Init?"=w463, "Prefix"=w462, "Current Gate"=w455, "Gate Name"=w465, "error in (no error)"=w464, "Image Characteristics"=w454, "Background Dataset"=w452) -> ("Init?"=w458:bool, "Dataset Images out"=w461:T25, "New Gate Image Refnum"=w460:T24, "Number of Created Images"=w457:i32, "error out"=w456:errorcluster)  [unwired: 2 in, 1 out]
                    n44 = call "AlliGator Image Pre-processing.vi"("Image Pre-Processing Parameters"=w459, "Data"=w468, "Buffer Image available?"=w458, "error in (no error)"=w456, "Current Gate"=w455, "Refnum in"=w460, "Dataset Images in"=w461) -> ("error out"=w467:errorcluster, "Dataset Images out"=w453:T25)  [unwired: 3 out]
                  }
                }
                n45 = Compound Arithmetic op=ADD(w418, w433, w447) -> (w448:i32)
                n46 = call "AlliGator Image Pre-processing.vi"("Image Pre-Processing Parameters"=w420, "Data"=w442, "Buffer Image available?"=w419, "error in (no error)"=w409, "Current Gate"=w417, "Refnum in"=w432, "Dataset Images in"=w431) -> ("error out"=w440:errorcluster, "Current Gate (dup)"=w434:i32, "# Replacements"=w446:i32, "Dataset Images out"=w436:T25, "Image Resolution"=w403:cluster{"X Resolution":i32, "Y Resolution":i32})
                n47 = Merge Errors(w440, w428) -> (w402:errorcluster)
                n48 = Unbundle By Name(w402) -> ("status"=w401:bool)
                n49 = Increment(x=w434) -> (x+1=w404:i32)
                n50 = Not(x=w401) -> (.not. x?=w400:bool)
                n51 = call "High Resolution Timing.vi"("relative seconds (NaN)"=w438, "Error In"=w402) -> ("elapsed (relative) seconds"=w437:dbl, "Error Out"=w439:errorcluster)  [unwired: 15 in, 1 out]
              }
              frame False {
                # "this gate mage is not used (e.g. skipped)\nor we are dealing with an already loaded background dataset"
              }
            }
            n52 = Compound Arithmetic op=AND(w316, w317) -> (w313:bool)
            n53 = case shown="True" w313 {
              tunnel: [_ w391] -> w361
              tunnel: w350 -> [w367 w390]
              tunnel: [w369 w389] -> w349
              tunnel: [w368 w388] -> w348
              tunnel: [w367 w387] -> w347
              tunnel: w340 -> [_ w386]
              tunnel: w339 -> [_ w385]
              tunnel: w336 -> [w363 w383]
              tunnel: [w363 w382] -> w335
              tunnel: w334 -> [_ w381]
              tunnel: w333 -> [_ w380]
              tunnel: w328 -> [w364 w379]
              tunnel: w327 -> [_ w377]
              tunnel: [w365 w376] -> w326
              tunnel: [w364 w375] -> w325
              tunnel: [w366 w374] -> w324
              tunnel: w323 -> [w369 w373]
              tunnel: w322 -> [w368 w372]
              tunnel: w321 -> [w366 w371]
              tunnel: w320 -> [w365 w370]
              frame False {
                # "if not done loading the gates, or \nnot reloading the background dataset"
              }
              frame True {
                # "Last step: updates shift register-stored data"
                n54 = call "AlliGator Last Gate Loading.vi"("Dataset Images 1 in"=w390, "Gates across boundaries?"=w385, "Split Index"=w386, "Dataset Images 2 in"=w379, "Current Gate"=w380, "VI in"=w381, "error in (no error)"=w383) -> ("Dataset Images 1 out"=w384:T25, "Dataset Images 2 out"=w378:T25, "# Disposed Images"=w391:i32, "error out"=w382:errorcluster)  [unwired: 5 in]
                n55 = case shown="True" w377 {
                  tunnel: [w395 w398] -> w388
                  tunnel: w384 -> [w394 w398]
                  tunnel: [w394 w399] -> w389
                  tunnel: w373 -> [_ w399]
                  tunnel: w372 -> [w395 _]
                  tunnel: [w394 w398] -> w387
                  tunnel: w378 -> [w393 w397]
                  tunnel: [w392 w397] -> w376
                  tunnel: [w393 w397] -> w375
                  tunnel: [w393 w396] -> w374
                  tunnel: w371 -> [_ w396]
                  tunnel: w370 -> [w392 _]
                  frame False {
                  }
                  frame True {
                  }
                }
              }
            }
          }
          n56 = case shown="True" w266 {
            tunnel: w269 -> [w306 w308]
            tunnel: [w306 w309] -> w268
            tunnel: w267 -> [_ w309]
            tunnel: w265 -> [w305 _]
            tunnel: [w305 w308] -> w264
            tunnel: [AlliGator_Variables_List."Files:Dataset Channel" ("Alligator Variable") AlliGator_Variables_List."Files:Background Dataset Channel" ("Alligator Variable")] -> w261
            frame False {
              # "Dataset"
            }
            frame True {
              # "background"
              # "Bkgd"
            }
          }
          n57 = call "Send Embedded Progress Bar Update.vi"("Stop Progress Bar (F)"=TRUE, "Progress Bar Queue in"=w248) -> ()  [unwired: 8 in, 2 out]
          n58 = Add Array Elements(numeric array=w284) -> (sum=w283:dbl)
          n59 = Add Array Elements(numeric array=w298) -> (sum=w297:i32)
          n60 = call "Get Common Image Resolution.vi"("Array of Image Resolutions"=w273) -> ("Y Resolution"=w271:i32, "X Resolution"=w272:i32)  [unwired: 8 in, 1 out]
          n61 = call "Number of Inf to NaN Conversions String.vi"("# Inf >> NaN"=w297) -> ("# inf >> NaN Conversion Sring"=w296:string)
          n62 = call "AlliGator Update Background File Subtraction Information.vi"("Background subtracted"=w281, "Error In"=w292, "Background Dataset Path"=w258, "Background Pixel Well Capacity"=w286, "Background Pile-up Correction"=w287) -> ("Error Out"=w263:errorcluster)  [unwired: 6 in]
          n63 = call "Alligator Variables Storage.vi"("Get(F)/Set"=TRUE, "AlliGator Variable"=w261, "Error In"=w263, "Data in"=w260) -> ("Error Out"=w255:errorcluster)  [unwired: 5 in, 2 out]
          n64 = call "Get File Name or Folder Name (wo .ext).vi"("error in (no error)"=w255, "input path"=w258) -> ("error out"=w254:errorcluster, "filename without extension"=w256:string, "dup path"=w257:path)  [unwired: 7 in]
        }
        frame Error {
        }
      }
      n65 = case shown="True" w181 {
        tunnel: w180 -> [_ w236]
        tunnel: [w224 w236] -> w140
        tunnel: w179 -> [w224 _]
        tunnel: w178 -> [w223 _]
        tunnel: [w223 w235] -> w177
        tunnel: w176 -> [_ w235]
        tunnel: w175 -> [w222 _]
        tunnel: w174 -> [_ w234]
        tunnel: [w222 w234] -> w173
        tunnel: w172 -> [w221 _]
        tunnel: [w221 w233] -> w171
        tunnel: w170 -> [_ w233]
        tunnel: w169 -> [_ w232]
        tunnel: [w220 w232] -> w168
        tunnel: w167 -> [w220 _]
        tunnel: w166 -> [_ w231]
        tunnel: [w219 w231] -> w165
        tunnel: w164 -> [w219 _]
        tunnel: w163 -> [w214 _]
        tunnel: [w214 w226] -> w162
        tunnel: w161 -> [w215 _]
        tunnel: [w215 w227] -> w160
        tunnel: w159 -> [w216 _]
        tunnel: [w216 w228] -> w158
        tunnel: w156 -> [w217 _]
        tunnel: [w217 w229] -> w157
        tunnel: w155 -> [_ w229]
        tunnel: w154 -> [w213 _]
        tunnel: [w213 w225] -> w153
        tunnel: w151 -> [w218 _]
        tunnel: [w218 w230] -> w150
        tunnel: w149 -> [_ w230]
        tunnel: w148 -> [_ w228]
        tunnel: w147 -> [_ w227]
        tunnel: w146 -> [_ w226]
        tunnel: w145 -> [_ w225]
        frame False {
          # "Image Dataset"
        }
        frame True {
          # "Background Dataset"
        }
      }
      n66 = call "AlliGator Update Dataset Series Slide.vi"("Dataset Series Slide Ref"=w137, "Current Time Stamp Ref"=w138, "Error In"=w139, "Path"=w140, "Dataset Series Paths"=w141, "Dataset Series Timestamps"=w142) -> ("Error Out"=w136:errorcluster, "Current Dataset"=w135:i32)  [unwired: 4 in]
      n67 = Select(t=w133, s=w136, f=w135) -> (s? t:f=w134:i32)
      n68 = in-place-cluster #2("Current Dataset"=w134, "Dual-Channel Background Dataset"=w183, "# Gates"=w150, "Background Dataset Images 1"=w173, "Current Dataset Images 1"=w168, "Background Dataset Images 2"=w171, "Current Dataset Images 2"=w165, "[Time-Series Timestamps]"=w142, "[Time-Series Paths]"=w141, "Single Data Point Path"=w140, "Current Folder"=w177, "Single Dataset Type"=w157, "I/m/phi Dataset.I/m/phi Dataset?"=w158, "Dual-Channel Dataset"=w160, "Channel Arithmetic"=w162, "Selected Channel Name"=w153) -> (w117:T23)
      n69 = property class="Str"(reference=w203, error in=w139, "Value"=w177) -> (error out=w202:errorcluster)  [unwired: 1 out]
    }
    n70 = in-place-dvr #1(w117) -> (→"Data Value Reference out":refnum<data-value>)  [unwired: 1 out]
  }
  "# Disposed Images" <- w86
  "# created images" <- w85
  "Dual-Channel Dataset" <- w33
  n71 = call "AlliGator Get ICCD Information.vi"("Y Resolution"=w1, "X Resolution"=w2, "Error In"=w7, "Y Software Binning"=w3, "X Software Binning"=w4, "File Info"=w9) -> ("Error Out"=w6:errorcluster, "ICCD-specific Information"=w8:T58)  [unwired: 4 in]
  n72 = case shown="True" w20 {
    tunnel: w89 -> [_ w544]
    tunnel: w79 -> [_ w542]
    tunnel: w78 -> [_ w541]
    tunnel: w76 -> [_ w540]
    tunnel: w75 -> [_ w537]
    tunnel: w74 -> [_ w536]
    tunnel: w73 -> [_ w535]
    tunnel: w72 -> [_ w534]
    tunnel: w66 -> [_ w533]
    tunnel: w65 -> [_ w532]
    tunnel: [w504 w531] -> w57
    tunnel: w52 -> [_ w530]
    tunnel: w48 -> [_ w526]
    tunnel: [w503 w525] -> w47
    tunnel: w5 -> [_ w524]
    tunnel: "selected path" -> [_ w523]
    tunnel: w44 -> [_ w522]
    tunnel: w4 -> [_ w521]
    tunnel: w3 -> [_ w520]
    tunnel: w32 -> [_ w519]
    tunnel: w30 -> [_ w518]
    tunnel: w29 -> [_ w517]
    tunnel: w2 -> [_ w516]
    tunnel: w1 -> [_ w515]
    tunnel: w27 -> [_ w514]
    tunnel: w26 -> [_ w513]
    tunnel: w24 -> [_ w512]
    tunnel: "Metadata" -> [_ w511]
    tunnel: "Data Description" -> [_ w510]
    tunnel: w21 -> [_ w509]
    tunnel: w6 -> [w504 w508]
    tunnel: w19 -> [w505 _]
    tunnel: w8 -> [_ w507]
    frame False {
      # "can be False if error or background file is unchanged"
      n73 = case shown="False" w505 {
        tunnel: ["Background Dataset unchanged (and not reloaded)" _] -> w503
        frame False {
          # "Background Dataset already loaded"
        }
        frame True {
          # "FLI Dataset & Error"
        }
      }
    }
    frame True {
      n74 = Bundle By Name(cluster=T59 {"Nanotime Gate Separation"=0.0, "Gate Width"=0.0, "Laser Period"=0.0, "Data Description"="", "# Pixel X"=0, "# Pixel Y"=0, "Gates to Use"={"Start"=0, "End"=0}, "Gate Step"=0, "SYNC Period"=0.0, "X Binning"=0, "Y Binning"=0, "Gates to"=FALSE, "Metadata"="", "Gate Image Exposure"=0.0, "Gate Image Integration"=0.0, "Macrotime Gate Separation"=0.0, "ICCD-specific Information"={"V MCP"=0.0, "X Hardware Binning"=0.0, "Y Hardware Binning"=0.0, "Gate Image Integration"=0.0, "Laser Power"=0.0}}, "X Binning"=w521, "Y Binning"=w520, "Gates to Use"=w517, "Gates to"=w533, "Nanotime Gate Separation"=w537, "Gate Width"=w540, "Laser Period"=w535, "# Pixel X"=w516, "# Pixel Y"=w515, "Gate Step"=w532, "Data Description"=w510, "SYNC Period"=w536, "Metadata"=w511, "Gate Image Exposure"=w514, "Gate Image Integration"=w513, "Macrotime Gate Separation"=w512, "ICCD-specific Information"=w507) -> (w528:T59)
      n75 = call "AlliGator Update Loaded Dataset Info.vi"("Image Loading Options"=w519, "Background File?"=w534, "Pile-up Correction"=w522, "error in (no error)"=w508, "After Loading Dataset Information"=w528, "# Gates"=w509, "Pixel Well Capacity"=w524) -> ("Error Out"=w529:errorcluster)  [unwired: 4 in]
      n76 = call "High Resolution Timing.vi"("relative seconds (NaN)"=w544, "Error In"=w529) -> ("elapsed (relative) seconds"=w539:dbl, "Error Out"=w538:errorcluster)  [unwired: 15 in, 1 out]
      n77 = Format Into String(format string="%s loaded: %s\n%s%s%s\n# Gates: %d\nLoad time: %#g s\nConversion time: %#g s\n", error in=w538, w541, w523, w526, w530, w518, w509, w539, w542) -> (resulting string=w525:string, error out=w531:errorcluster)  [unwired: 1 in]
    }
  }
  "error out" <- w57
  "Message" <- w47
  n78 = call "Set Slide Range.vi"("Max"=w21, "error in (no error)"=w7, "Slide in"=w56) -> ("error out"=w59:errorcluster)  [unwired: 8 in]
  n79 = Merge Errors(w59, w60) -> (w58:errorcluster)
  n80 = call "Clear Error.vi"("Error In"=w58) -> ()  [unwired: 8 in, 1 out]
